vi "Create Channel.vi"(6 "index":i32, 8 "error in":errorcluster, 10 "channel settings":T1, 11 "digital input mode in":refnum<class "Digital Input Mode.lvclass">) -> (0 "error out":errorcluster, 2 "digital input channel":refnum<class "DI Channel.lvclass">, 3 "digital input mode out":refnum<class "Digital Input Mode.lvclass">)   [LabVIEW 2020, in "Scan Engine Scripting.lvlib" / "Digital Input Mode.lvclass"]
uses:
  Digital Input Mode.lvclass
  Controls/digital channel settings.ctl
  Channel Classes/DI Channel/DI Channel.lvclass
  Digital Input Mode.lvclass/Digital Input Mode.ctl
  Scan Engine Scripting.lvlib
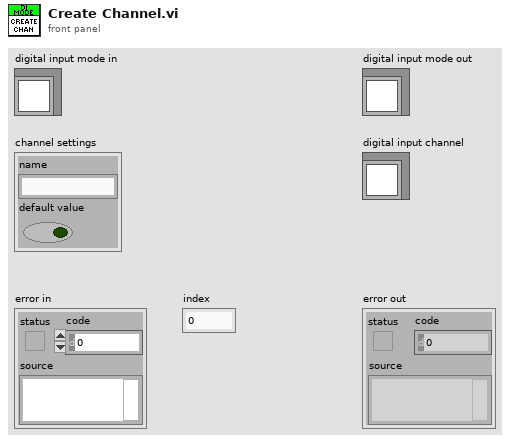
[diagram p1: front panel]
types:
  T1 = typedef "Scan Engine Scripting.lvlib/digital channel settings.ctl" = cluster{"name":string, "default value":bool}
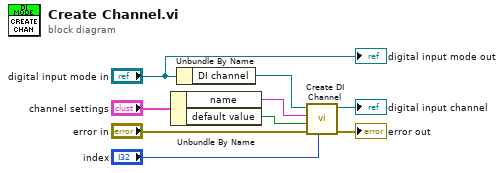
[diagram p0: block diagram]
diagram:
  n1 = Unbundle By Name("channel settings") -> ("name"=w1:string, "default value"=w2:bool)
  n2 = Unbundle By Name("digital input mode in") -> ("DI channel"=w3:refnum<class "DI Channel.lvclass">)
  n3 = call "Create DI Channel.vi"("index"="index", "error in"="error in", "default value"=w2, "name"=w1, "DI channel in"=w3) -> ("error out"=→"error out":errorcluster, "DI channel out"=→"digital input channel":refnum<class "DI Channel.lvclass">)  [unwired: 5 in]
  "digital input mode out" <- "digital input mode in"
